vi "conexionLabviewEJS.vi"() -> ()   [LabVIEW 2010]
panel:
  in  "stop":bool
  out "intind":i32
  in  "intcon":i32
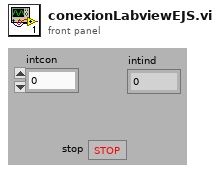
[diagram p1: front panel]
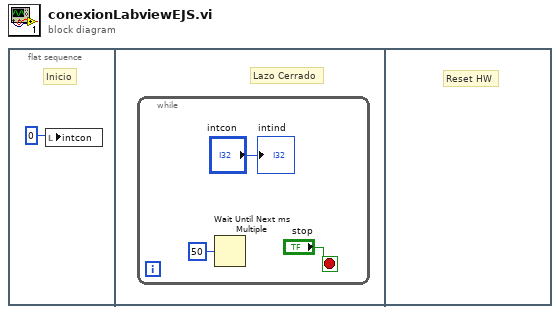
[diagram p0: block diagram]
diagram:
  n1 = flat-sequence {
    frame #0 {
      # "Inicio"
      n2 = local write "intcon"(i16 0 ("int_con")) -> ()
    }
    frame #1 {
      # "Lazo Cerrado"
      n3 = while {
        stop <- "stop" stop-if-true
        n4 = Wait Until Next ms Multiple(millisecond multiple=u32 50) -> ()  [unwired: 1 out]
        "intind" <- "intcon"
      }
    }
    frame #2 {
      # "Reset HW"
    }
  }
